vi "Draw Joint.vi"(4 "Body Index":i32, 6 "Color":u32(colorbox)=16711680, 7 "Include Inferred Joints?":bool=TRUE, 8 "error in":errorcluster, 9 "JointType":T2 items=["SpineBase", "SpineMid", "Neck", "Head", "ShoulderLeft", "ElbowLeft", "WristLeft", "HandLeft", "ShoulderRight", "ElbowRight", "WristRight", "HandRight", "HipLeft", "KneeLeft", "AnkleLeft", "FootLeft", "HipRight", "KneeRight", "AnkleRight", "FootRight", "SpineShoulder", "HandTipLeft", "ThumbLeft", "HandTipRight", "ThumbRight"], 11 "Image":T1) -> (0 "error out":errorcluster, 3 "Image Out":T1)   [LabVIEW 2014]
uses:
  controls/JointType.ctl
  <vilib>/vision/Image Controls.llb/IMAQ Image.ctl
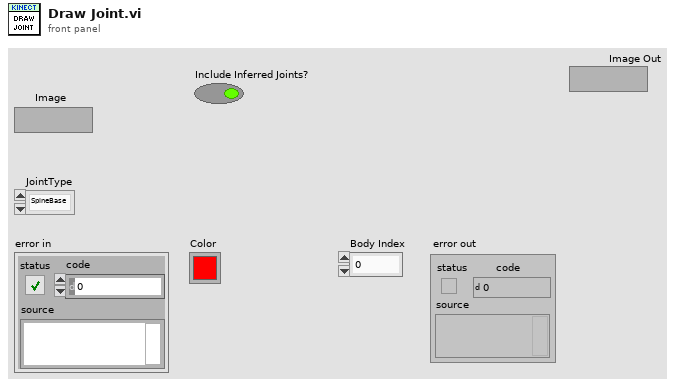
[diagram p1: front panel]
types:
  T1 = typedef "IMAQ Image.ctl" = refnum<image>
  T2 = typedef "JointType.ctl" = i32
  T3 = typedef "Joint Position.ctl" = cluster{"Position":cluster{"X":sgl, "Y":sgl}, "TrackingState":i32}
  T4 = cluster{"Left":i32, "Top":i32, "Right":i32, "Bottom":i32}
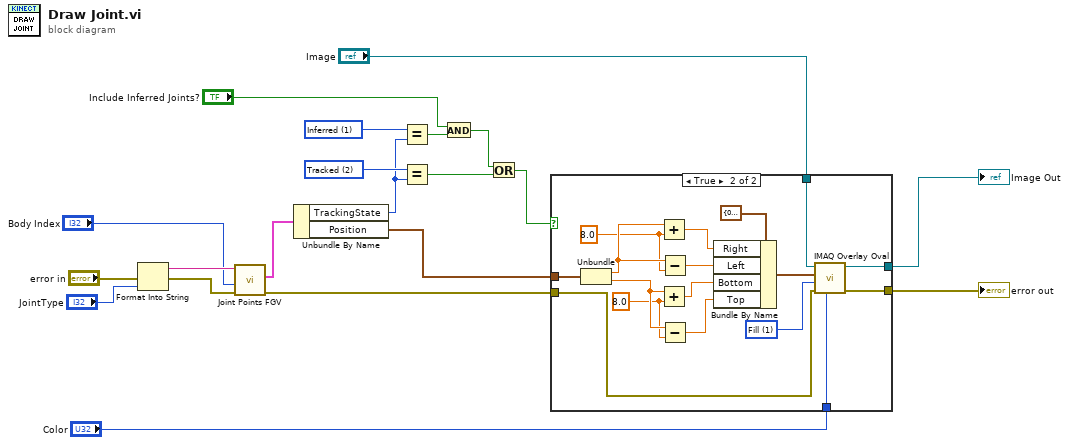
[diagram p0: block diagram]
diagram:
  w7 = 1 items=["NotTracked", "Inferred", "Tracked"] ("TrackingState")
  w8 = 2 items=["NotTracked", "Inferred", "Tracked"] ("TrackingState")
  n1 = Format Into String(error in="error in", "JointType") -> (resulting string=w19:string, error out=w18:errorcluster)  [unwired: 2 in]
  n2 = call "Joint Points FGV.vi"("error in (no error)"=w18, "Body Index"="Body Index", "name"=w19) -> ("error out"=w13:errorcluster, "Joint Position"=w10:T3)  [unwired: 7 in]
  n3 = Unbundle By Name(w10) -> ("TrackingState"=w6:i32, "Position"=w9:cluster{"X":sgl, "Y":sgl})
  n4 = Equal?(x=w7, y=w6) -> (x = y?=w5:bool)
  n5 = Equal?(x=w8, y=w6) -> (x = y?=w2:bool)
  n6 = And(x="Include Inferred Joints?", y=w5) -> (x .and. y?=w3:bool)
  n7 = Or(x=w3, y=w2) -> (x .or. y?=w1:bool)
  n8 = case shown="True" w1 {
    tunnel: "Image" -> [w22 w29]
    tunnel: [w22 w28] -> w16
    tunnel: [w21 w27] -> w15
    tunnel: w13 -> [w21 w25]
    tunnel: "Color" -> [_ w24]
    tunnel: w9 -> [_ w23]
    frame False {
    }
    frame True {
      w26 = u32 1 items=["Frame", "Fill"] ("Drawing Mode (Frame)")
      w33 = sgl 8.0 ("y")
      w37 = sgl 8.0 ("y")
      n9 = Unbundle(w23) -> ("X"=w38:sgl, "Y"=w34:sgl)
      n10 = Add(x=w38, y=w37) -> (x+y=w36:sgl)
      n11 = Add(x=w34, y=w33) -> (x+y=w32:sgl)
      n12 = Subtract(x=w38, y=w37) -> (x-y=w35:sgl)
      n13 = Subtract(x=w34, y=w33) -> (x-y=w31:sgl)
      n14 = Bundle By Name(cluster=T4 {"Left"=0, "Top"=0, "Right"=0, "Bottom"=0} ("Bounding Rectangle"), "Right"=w36, "Left"=w35, "Bottom"=w32, "Top"=w31) -> (w30:T4)
      n15 = call "IMAQ Overlay Oval"("Color"=w24, "error in (no error)"=w25, "Drawing Mode (Frame)"=w26, "Bounding Rectangle"=w30, "Image"=w29) -> ("error out"=w27:errorcluster, "Image Out"=w28:T1)  [unwired: 5 in]
    }
  }
  "Image Out" <- w16
  "error out" <- w15
